vi "sizes.vi"(8 "Size 4":i32, 9 "Size 3":i32, 10 "Size 2":i32, 11 "Size 1":i32) -> (0 "led 2":i32, 1 "led 1":i32, 3 "Problem":bool)   [LabVIEW 2011]
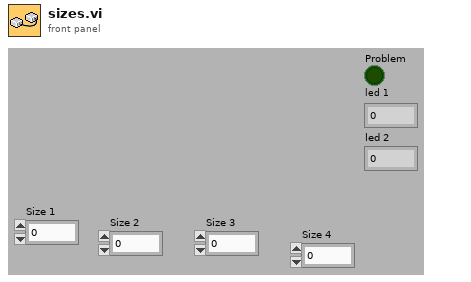
[diagram p1: front panel]
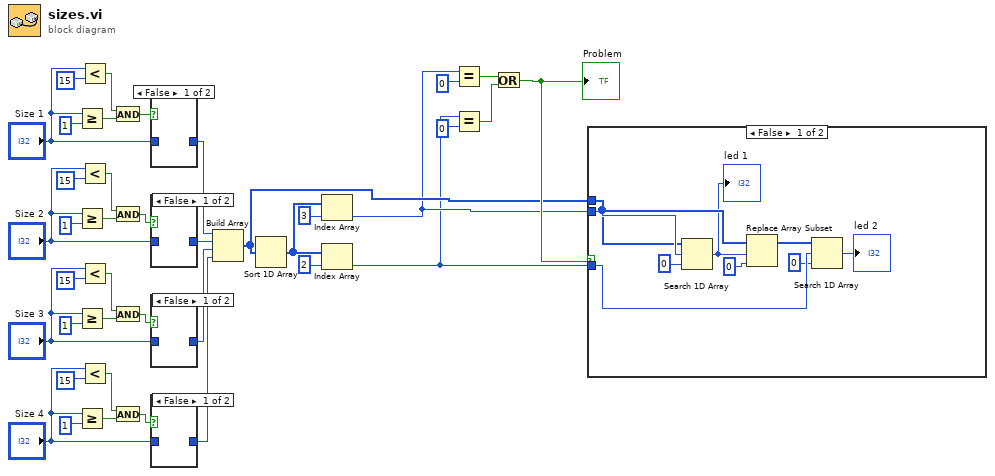
[diagram p0: block diagram]
diagram:
  n1 = Greater Or Equal?(x="Size 1", y=1) -> (x >= y?=w36:bool)
  n2 = Greater Or Equal?(x="Size 2", y=1) -> (x >= y?=w32:bool)
  n3 = Greater Or Equal?(x="Size 3", y=1) -> (x >= y?=w28:bool)
  n4 = Greater Or Equal?(x="Size 4", y=1) -> (x >= y?=w24:bool)
  n5 = Less?(x="Size 1", y=15) -> (x < y?=w37:bool)
  n6 = Less?(x="Size 2", y=15) -> (x < y?=w33:bool)
  n7 = Less?(x="Size 3", y=15) -> (x < y?=w29:bool)
  n8 = Less?(x="Size 4", y=15) -> (x < y?=w25:bool)
  n9 = And(x=w37, y=w36) -> (x .and. y?=w23:bool)
  n10 = And(x=w33, y=w32) -> (x .and. y?=w20:bool)
  n11 = And(x=w29, y=w28) -> (x .and. y?=w13:bool)
  n12 = And(x=w25, y=w24) -> (x .and. y?=w12:bool)
  n13 = case shown="False" w23 {
    tunnel: "Size 1" -> [_ w40]
    tunnel: [_ w40] -> w21
    frame False {
    }
    frame True {
    }
  }
  n14 = case shown="False" w20 {
    tunnel: "Size 2" -> [_ w41]
    tunnel: [_ w41] -> w18
    frame False {
    }
    frame True {
    }
  }
  n15 = case shown="False" w13 {
    tunnel: "Size 3" -> [_ w42]
    tunnel: [_ w42] -> w15
    frame False {
    }
    frame True {
    }
  }
  n16 = case shown="False" w12 {
    tunnel: "Size 4" -> [_ w43]
    tunnel: [_ w43] -> w14
    frame False {
    }
    frame True {
    }
  }
  n17 = Build Array(w21, w18, w15, w14) -> (w3:i32[])
  n18 = Sort 1D Array(array=w3) -> (sorted array=w11:i32[])
  n19 = Index Array(array=w11, index=3) -> (element=w2:i32)
  n20 = Index Array(array=w11, index=2) -> (element=w1:i32)
  n21 = Equal?(x=w2, y=0) -> (x = y?=w6:bool)
  n22 = Equal?(x=w1, y=0) -> (x = y?=w5:bool)
  n23 = Or(x=w6, y=w5) -> (x .or. y?=w4:bool)
  "Problem" <- w4
  n24 = case shown="False" w4 {
    tunnel: w3 -> [w47 _]
    tunnel: w2 -> [w52 _]
    tunnel: w1 -> [w50 _]
    frame False {
      n25 = Search 1D Array(1D array=w47, element=w52, start index (0)=0) -> (index of element=w46:i32)
      "led 1" <- w46
      n26 = Replace Array Subset(array=w47, new element=0 ("new element/subarray"), index=w46) -> (w44:i32[])
      n27 = Search 1D Array(1D array=w44, element=w50, start index (0)=0) -> (index of element=→"led 2":i32)
    }
    frame True {
    }
  }
